vi "Log_MessageHanlder_CountMessagesInLogFile.vi"(8 "error in":errorcluster, 11 "MessageHandler in":refnum<class "MessageHandler.lvclass">) -> (0 "error out":errorcluster, 2 "NbMessages":i32, 3 "MessageHandler out":refnum<class "MessageHandler.lvclass">)   [LabVIEW 2013, in "MessageHandler.lvclass"]
uses:
  MessageHandler.lvclass
  030 - EVENTS/03 - ToMessageHandlerProcess/ToMessageHandlerEvent.ctl
  030 - EVENTS/03 - ToMessageHandlerProcess/enumMessageCriticity.ctl
  MessageHandler.lvclass/MessageHandler.ctl
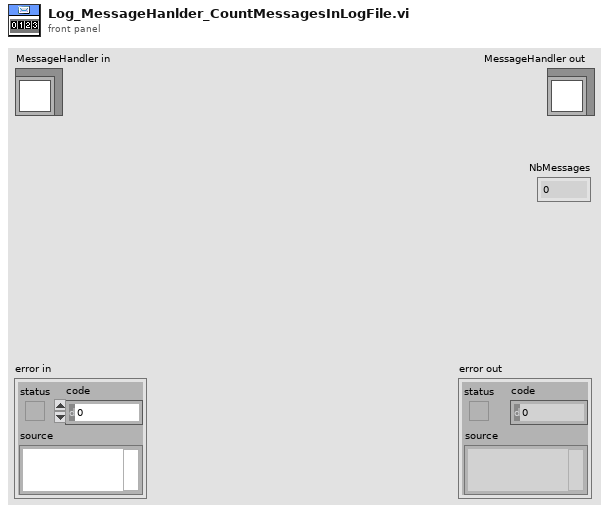
[diagram p1: front panel]
types:
  T1 = enum16{"open", "replace", "create", "open or create", "replace or create", "replace or create with confirmation"}
  T2 = typedef "ToMessageHandlerEvent.ctl" = cluster{"date / time":timestamp, "Criticity":T3, "Emitter":string, "Message":string}
  T3 = typedef "enumMessageCriticity.ctl" = enum16{"No error", "Info", "Warning", "Error", "Fatal error"}
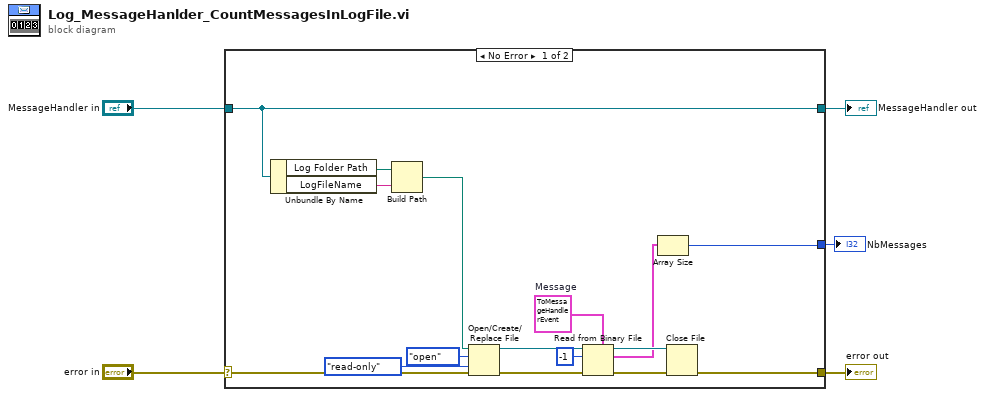
[diagram p0: block diagram]
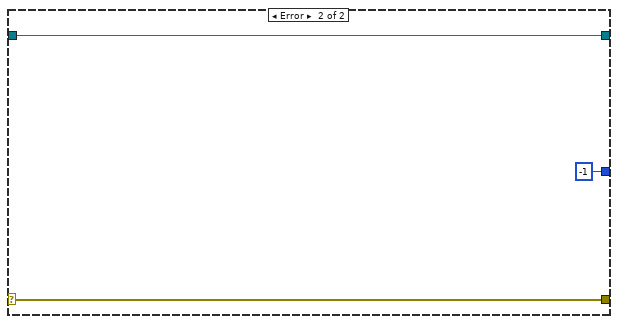
[diagram p2: hidden frame]
diagram:
  n1 = case shown="No Error" "error in" {
    selector: "error in" -> [w17 w24]
    tunnel: [w9 w24] -> w4
    tunnel: [w21 w23] -> w2
    tunnel: "MessageHandler in" -> [w21 w23]
    tunnel: [w6 -1] -> w1
    frame No Error {
      w14 = T2 {"date / time"=timestamp(0 s since 1904-01-01), "Criticity"=enum."No error", "Emitter"="", "Message"=""}  # Message
      n2 = Unbundle By Name(w21) -> ("Log Folder Path"=w20:path, "LogFileName"=w19:string)
      n3 = Build Path(base path=w20, name or relative path=w19) -> (appended path=w18:path)
      n4 = Open/Create/Replace File(file path (use dialog)=w18, error in=w17, operation (0:open)=T1."open", access (0:read/write)=enum16{"read/write", "read-only", "write-only"}."read-only") -> (refnum out=w12:refnum<file>, error out=w11:errorcluster)  [unwired: 2 in, 1 out]
      n5 = Read from Binary File(5:w14, 8:w11, 10:-1 ("count (1)"), 11:w12) -> (0:w10:errorcluster, 2:w7:T2[], 3:w8:refnum<file>)  [unwired: 2 in, 1 out]
      n6 = Array Size(array=w7) -> (size(s)=w6:i32)
      n7 = Close File(refnum=w8, error in=w10) -> (error out=w9:errorcluster)  [unwired: 1 out]
    }
    frame Error {
    }
  }
  "error out" <- w4
  "MessageHandler out" <- w2
  "NbMessages" <- w1
